vi "Perform Step.vi"(8 "error in (no error)":errorcluster, 9 "Keyboard":refnum<k1>, 10 "Hotkeys":T1, 11 "Step":T2={"Type"=enum."Mouse Move", "X"=0, "Y"=0, "Delay"=0, "Key"=65, "Repeat"=0, "RClick?"=FALSE, "App/Window Name"="", "Notes"=""}) -> (0 "error out":errorcluster, 3 "State(s)":string)   [LabVIEW 2023]
doc: "Executes <B>Step</B>, checks for an abort hotkey press, and outputs the next state for the state machine to execute based on the step and <B>Repeat Count</B>."
uses:
  ec44d10e-72d8-4c7e-b1c7-11b5471dc187.vi
  CTLs/Hotkey Type.ctl
  CTLs/FGV Actions.ctl
  labview_win_util32_8.6/Winevent/Winevent.lvlib
  labview_win_util32_8.6/WINUTIL/WINUTIL.lvlib
  0fc491d1-540b-4e3c-a9f1-d515ab3959d5.vi
  eed0c13c-4c8d-4811-bf1b-886c68460aaa.vi
  27aa0f71-d9e0-4e00-a40a-04ebf7167400.vi
  70c2b0c9-e855-47dc-a99c-854f52cf3209.vi
  2266d4d6-2cac-4868-b53d-76dc73e57a79.vi
  f6af166c-5c2a-40ab-b52b-e7588615a589.vi
  1d40764d-0ee2-42e1-b1e2-1dce413207b4.vi
  CTLs/Step Type V3.ctl
  CTLs/Hotkey Values.ctl
  CTLs/Step V3.ctl
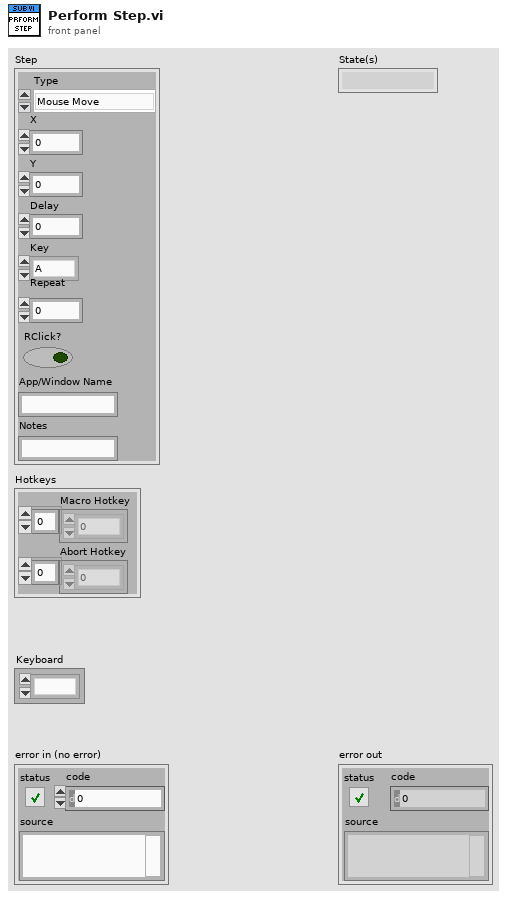
[diagram p1: front panel]
types:
  T1 = typedef "Hotkey Values.ctl" = cluster{"Macro Hotkey":enum16{"0", "1", "2", "3", "4", "5", "6", "7", "8", "9", "A", "B", "C", "D", "E", "F", "G", "H", "I", "J", "K", "L", "M", "N", "O", "P", "Q", "R", "S", "T", "U", "V", "W", "X", "Y", "Z", "F1", "F2", "F3", "F4", "F5", "F6", "F7", "F8", "F9", "F10", "F11", "F12", "F13", "F14", "F15", "ADD", "BACK", "BACKSLASH", "CAPITAL", "COMMA", "DECIMAL", "DELETE", "DIVIDE", "DOWN", "END", "EQUALS", "ESCAPE", "GRAVE (`)", "HOME", "INSERT", "LBRACKET", "LCONTROL", "LEFT", "L ALT", "LSHIFT", "LWIN", "MINUS", "MULTIPLY", "NEXT", "NUMLOCK", "NUMPAD_0", "NUMPAD_1", "NUMPAD_2", "NUMPAD_3", "NUMPAD_4", "NUMPAD_5", "NUMPAD_6", "NUMPAD_7", "NUMPAD_8", "NUMPAD_9", "PAUSE", "PERIOD", "PRIOR (PG UP)", "RBRACKET", "RCONTROL", "RETURN", "RIGHT", "R ALT", "RSHIFT", "RWIN", "SCROLL", "SEMICOLON", "SLASH", "SPACE", "SUBTRACT", "TAB", "UP", "ENTER (num pad)", "' (quote)"}[], "Abort Hotkey":enum16{"0", "1", "2", "3", "4", "5", "6", "7", "8", "9", "A", "B", "C", "D", "E", "F", "G", "H", "I", "J", "K", "L", "M", "N", "O", "P", "Q", "R", "S", "T", "U", "V", "W", "X", "Y", "Z", "F1", "F2", "F3", "F4", "F5", "F6", "F7", "F8", "F9", "F10", "F11", "F12", "F13", "F14", "F15", "ADD", "BACK", "BACKSLASH", "CAPITAL", "COMMA", "DECIMAL", "DELETE", "DIVIDE", "DOWN", "END", "EQUALS", "ESCAPE", "GRAVE (`)", "HOME", "INSERT", "LBRACKET", "LCONTROL", "LEFT", "L ALT", "LSHIFT", "LWIN", "MINUS", "MULTIPLY", "NEXT", "NUMLOCK", "NUMPAD_0", "NUMPAD_1", "NUMPAD_2", "NUMPAD_3", "NUMPAD_4", "NUMPAD_5", "NUMPAD_6", "NUMPAD_7", "NUMPAD_8", "NUMPAD_9", "PAUSE", "PERIOD", "PRIOR (PG UP)", "RBRACKET", "RCONTROL", "RETURN", "RIGHT", "R ALT", "RSHIFT", "RWIN", "SCROLL", "SEMICOLON", "SLASH", "SPACE", "SUBTRACT", "TAB", "UP", "ENTER (num pad)", "' (quote)"}[]}
  T2 = typedef "Step V3.ctl" = cluster{"Type":T3, "X":i32, "Y":i32, "Delay":i32, "Key":u8, "Repeat":i32, "RClick?":bool, "App/Window Name":string, "Notes":string}
  T3 = typedef "Step Type V3.ctl" = enum16{"Mouse Move", "Mouse Click", "Key Press", "Wait", "Mouse Down", "Mouse Up", "Key Down", "Key Up", "Run Application", "Maximize Window", "Restore Window", "Minimize Window", "Close Window", "Bring Window to Front", "Send Window to Back"}
  T4 = typedef "Hotkey Type.ctl" = enum16{"Macro Hotkey", "Abort Hotkey"}
  T5 = typedef "FGV Actions.ctl" = enum16{"Read", "Write"}
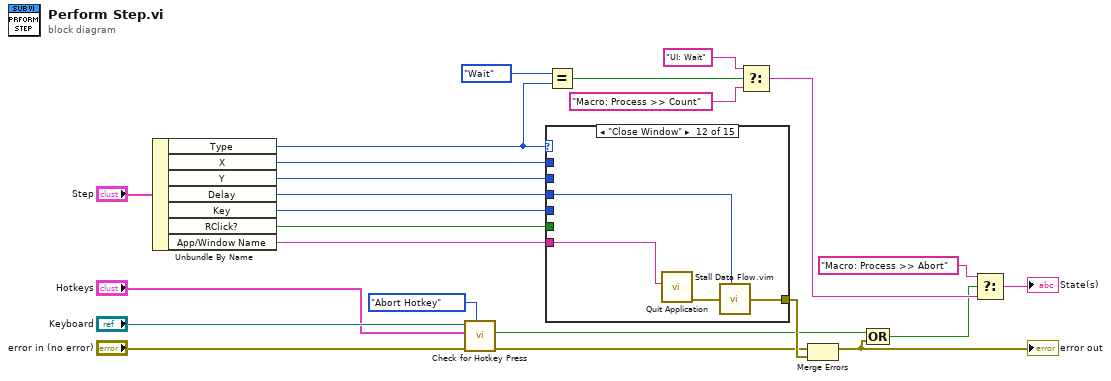
[diagram p0: block diagram]
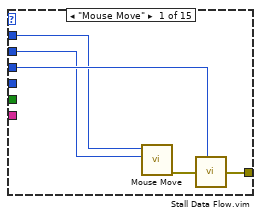
[diagram p2: hidden frame]
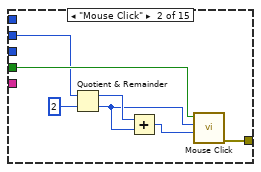
[diagram p3: hidden frame]
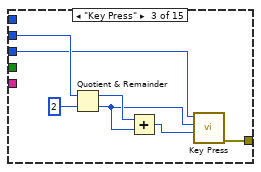
[diagram p4: hidden frame]
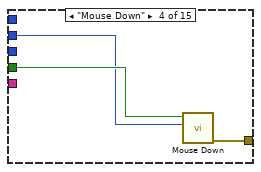
[diagram p5: hidden frame]
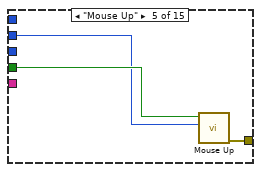
[diagram p6: hidden frame]
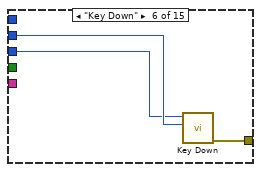
[diagram p7: hidden frame]
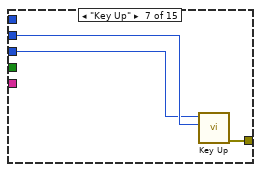
[diagram p8: hidden frame]
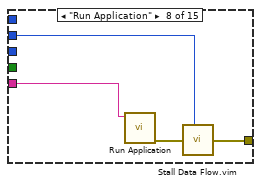
[diagram p9: hidden frame]
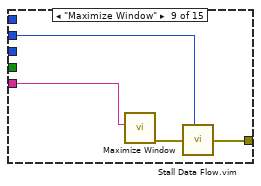
[diagram p10: hidden frame]
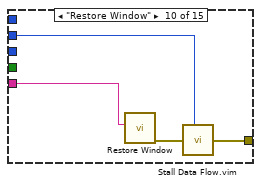
[diagram p11: hidden frame]
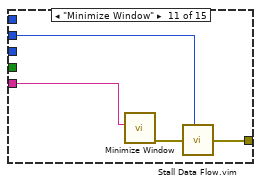
[diagram p12: hidden frame]
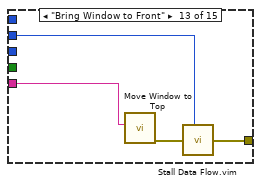
[diagram p13: hidden frame]
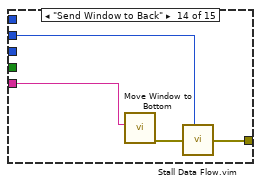
[diagram p14: hidden frame]
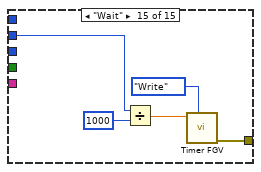
[diagram p15: hidden frame]
diagram:
  n1 = Unbundle By Name("Step") -> ("Type"=w3:T3, "X"=w24:i32, "Y"=w6:i32, "Delay"=w23:i32, "Key"=w22:u8, "RClick?"=w21:bool, "App/Window Name"=w7:string)
  n2 = call "Check for Hotkey Press.vi"("Hotkey Type"=Hotkey_Type."Abort Hotkey", "error in (no error)"="error in (no error)", "Hotkeys"="Hotkeys", "Keyboard"="Keyboard") -> ("error out"=w12:errorcluster, "Pressed?"=w10:bool)  [unwired: 5 in, 1 out]
  n3 = case shown="\"Close Window\"" w3 {
    tunnel: w24 -> [w26 _ _ _ _ _ _ _ _ _ _ _ _ _ _]
    tunnel: w23 -> [w27 w34 w42 w44 w47 w51 w54 w56 w60 w64 w68 w72 w76 w80 w88]
    tunnel: w22 -> [_ _ w37 _ _ w50 w53 _ _ _ _ _ _ _ _]
    tunnel: [w28 w36 w43 w46 w49 w52 w55 w57 w61 w65 w69 w73 w77 w81 w85] -> w13
    tunnel: w21 -> [_ w35 _ w45 w48 _ _ _ _ _ _ _ _ _ _]
    tunnel: w7 -> [_ _ _ _ _ _ _ w58 w62 w66 w70 w74 w78 w82 _]
    tunnel: w6 -> [w25 _ _ _ _ _ _ _ _ _ _ _ _ _ _]
    frame "Mouse Move" {
      n4 = call "Mouse Move.vi"("y"=w25, "x"=w26) -> ("error out"=w29:errorcluster)  [unwired: 9 in]
      n5 = call "Stall Data Flow.vim"("value in"=w29, "milliseconds to wait"=w27) -> ("value out"=w28:errorcluster)  [unwired: 1 out]
    }
    frame "Mouse Click" {
      n6 = Quotient & Remainder(x=w34, y=2) -> (x-y*floor(x/y)=w32:i32, floor(x/y)=w30:i32)
      n7 = Add(x=w32, y=w30) -> (x+y=w31:i32)
      n8 = call "Mouse Click.vi"("ms wait after up (10)"=w31, "ms wait after down (10)"=w30, "Right Click? (F)"=w35) -> ("error out"=w36:errorcluster)  [unwired: 8 in]
    }
    frame "Key Press" {
      n9 = Quotient & Remainder(x=w42, y=2) -> (x-y*floor(x/y)=w40:i32, floor(x/y)=w38:i32)
      n10 = Add(x=w40, y=w38) -> (x+y=w39:i32)
      n11 = call "Key Press.vi"("ms wait after up (20)"=w39, "ms wait after down (80)"=w38, "Virtual Key"=w37) -> ("error out"=w43:errorcluster)  [unwired: 8 in]
    }
    frame "Mouse Down" {
      n12 = call "Mouse Down.vi"("Delay in ms (10)"=w44, "Right Click? (F)"=w45) -> ("error out"=w46:errorcluster)  [unwired: 9 in]
    }
    frame "Mouse Up" {
      n13 = call "Mouse Up.vi"("Delay in ms (10)"=w47, "Right Click? (F)"=w48) -> ("error out"=w49:errorcluster)  [unwired: 9 in]
    }
    frame "Key Down" {
      n14 = call "Key Down.vi"("delay in ms (80)"=w51, "Virtual Key"=w50) -> ("error out"=w52:errorcluster)  [unwired: 9 in]
    }
    frame "Key Up" {
      n15 = call "Key Up.vi"("delay in ms (20)"=w54, "Virtual Key"=w53) -> ("error out"=w55:errorcluster)  [unwired: 9 in]
    }
    frame "Run Application" {
      n16 = call "Run Application.vi"("command line to execute (\"\")"=w58) -> ("error out"=w59:errorcluster)  [unwired: 9 in, 1 out]
      n17 = call "Stall Data Flow.vim"("value in"=w59, "milliseconds to wait"=w56) -> ("value out"=w57:errorcluster)  [unwired: 1 out]
    }
    frame "Maximize Window" {
      n18 = call "Maximize Window.vi"("window name  (\"\")"=w62) -> ("error out"=w63:errorcluster)  [unwired: 5 in, 1 out]
      n19 = call "Stall Data Flow.vim"("value in"=w63, "milliseconds to wait"=w60) -> ("value out"=w61:errorcluster)  [unwired: 1 out]
    }
    frame "Restore Window" {
      n20 = call "Restore Window.vi"("window name  (\"\")"=w66) -> ("error out"=w67:errorcluster)  [unwired: 5 in, 1 out]
      n21 = call "Stall Data Flow.vim"("value in"=w67, "milliseconds to wait"=w64) -> ("value out"=w65:errorcluster)  [unwired: 1 out]
    }
    frame "Minimize Window" {
      n22 = call "Minimize Window.vi"("window name  (\"\")"=w70) -> ("error out"=w71:errorcluster)  [unwired: 5 in, 1 out]
      n23 = call "Stall Data Flow.vim"("value in"=w71, "milliseconds to wait"=w68) -> ("value out"=w69:errorcluster)  [unwired: 1 out]
    }
    frame "Close Window" {
      n24 = call "Quit Application.vi"("window name (\"\")"=w74) -> ("error out"=w75:errorcluster)  [unwired: 10 in]
      n25 = call "Stall Data Flow.vim"("value in"=w75, "milliseconds to wait"=w72) -> ("value out"=w73:errorcluster)  [unwired: 1 out]
    }
    frame "Bring Window to Front" {
      n26 = call "Move Window to Top.vi"("window name (\"\")"=w78) -> ("error out"=w79:errorcluster)  [unwired: 5 in, 1 out]
      n27 = call "Stall Data Flow.vim"("value in"=w79, "milliseconds to wait"=w76) -> ("value out"=w77:errorcluster)  [unwired: 1 out]
    }
    frame "Send Window to Back" {
      n28 = call "Move Window to Bottom.vi"("window name (\"\")"=w82) -> ("error out"=w83:errorcluster)  [unwired: 5 in, 1 out]
      n29 = call "Stall Data Flow.vim"("value in"=w83, "milliseconds to wait"=w80) -> ("value out"=w81:errorcluster)  [unwired: 1 out]
    }
    frame "Wait" {
      n30 = Divide(x=w88, y=1000) -> (x/y=w84:dbl)
      n31 = call "Timer FGV.vi"("Mode"=FGV_Actions."Write", "Timer Value (s)"=w84) -> ("error out"=w85:errorcluster)  [unwired: 7 in, 2 out]
    }
  }
  n32 = Equal?(x=Step_Type_V3."Wait", y=w3) -> (x = y?=w1:bool)
  n33 = Select(t="UI: Wait", s=w1, f="Macro: Process >> Count") -> (s? t:f=w9:string)
  n34 = Merge Errors(w12, w13) -> (w17:errorcluster)
  "error out" <- w17
  n35 = Compound Arithmetic op=OR(w10, w17) -> (w8:bool)
  n36 = Select(t="Macro: Process >> Abort", s=w8, f=w9) -> (s? t:f=→"State(s)":string)
